vi "Read DMM - Current Mode.vi"(8 "error in (no error)":errorcluster, 11 "Async Data in":T1={"Hardware"={"Switch Device"="", "DMM Device"="", "DMM -> Switch Trigger"=0, "Switch -> DMM Trigger"=0, "Sample Interval (sec)"=0.0, "Current Samples"=0, "Current Limit"=1.2, "Current Resolution"=5.5, "Auto-Read"=FALSE, "Keep Values"=FALSE}, "Communication"={"Status Q"=refnum, "Command Q"=refnum, "Voltage FIFO"=refnum, "Voltage Buffer"=[], "Current FIFO"=refnum, "Current Buffer"=[], "Async Events"=refnum}} {"Hardware"."Current Resolution" items=["3 1/2"=3.5, "4 1/2"=4.5, "5 1/2"=5.5, "6 1/2"=6.5, "7 1/2"=7.5]; "Hardware"."Sample Interval (sec)" format="%.2f"}) -> (0 "error out":errorcluster, 3 "Acquiring":bool)   [LabVIEW 2011, in "Switch-DMM Custom Device.lvlib"]
uses:
  Switch-DMM Custom Device.lvlib
  Controls/Async Data.ctl
  Controls/Hardware.ctl
  <instrlib>/niDMM/nidmm.llb/niDMM Resolution in Digits.ctl
  Controls/Communication.ctl
  Controls/Async Status.ctl
  Controls/Async State.ctl
  Controls/Async Command.ctl
  Controls/Async Events.ctl
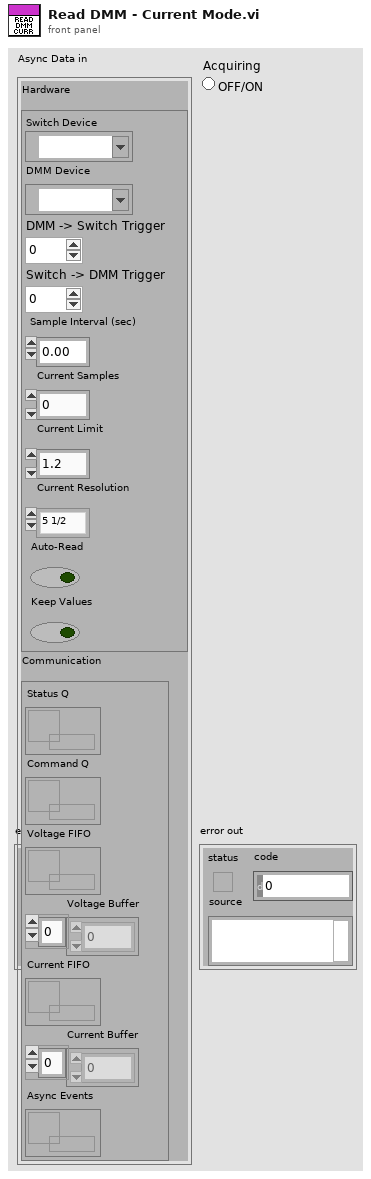
[diagram p1: front panel]
types:
  T1 = typedef "Switch-DMM Custom Device.lvlib/Async Data.ctl" = cluster{"Hardware":T2, "Communication":T4}
  T2 = typedef "Switch-DMM Custom Device.lvlib/Hardware.ctl" = cluster{"Switch Device":refnum<k15>, "DMM Device":refnum<k15>, "DMM -> Switch Trigger":u16, "Switch -> DMM Trigger":u16, "Sample Interval (sec)":dbl, "Current Samples":i32, "Current Limit":dbl, "Current Resolution":T3, "Auto-Read":bool, "Keep Values":bool}
  T3 = typedef "niDMM Resolution in Digits.ctl" = dbl
  T4 = typedef "Switch-DMM Custom Device.lvlib/Communication.ctl" = cluster{"Status Q":refnum<queue>, "Command Q":refnum<queue>, "Voltage FIFO":refnum<k33>, "Voltage Buffer":dbl[], "Current FIFO":refnum<k33>, "Current Buffer":dbl[], "Async Events":refnum<queue>}
  T5 = typedef "Switch-DMM Custom Device.lvlib/Async Events.ctl" = enum16{"None", "Over Current", "Volt Read Done"}
  T6 = typedef "Switch-DMM Custom Device.lvlib/Async Command.ctl" = enum16{"None", "Start", "Set Cur Mode", "Req Volt Mode", "Set Volt Mode", "Read Volt", "Exit"}
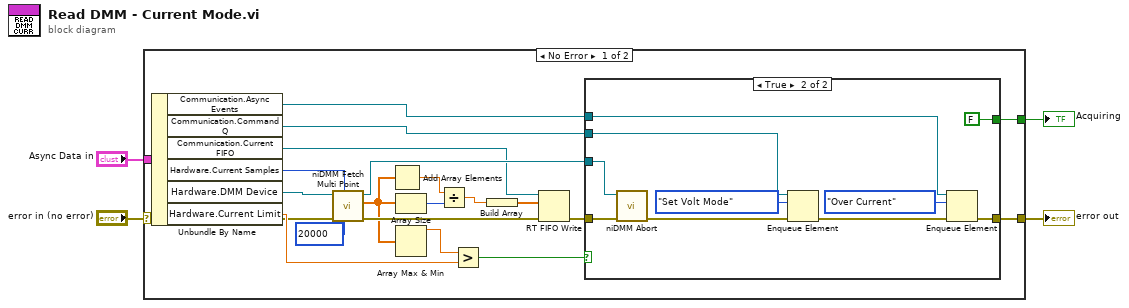
[diagram p0: block diagram]
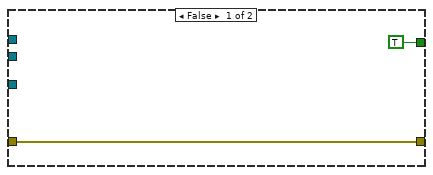
[diagram p2: hidden frame]
diagram:
  n1 = case shown="No Error" "error in (no error)" {
    selector: "error in (no error)" -> [w15 w38]
    tunnel: [w21 w38] -> w4
    tunnel: [w20 _] -> w3
    tunnel: "Async Data in" -> [w16 _]
    frame No Error {
      n2 = Unbundle By Name(w16) -> ("Communication.Async Events"=w13:refnum<queue>, "Communication.Command Q"=w14:refnum<queue>, "Communication.Current FIFO"=w12:refnum<k33>, "Hardware.Current Samples"=w11:i32, "Hardware.DMM Device"=w19:refnum<k15>, "Hardware.Current Limit"=w22:dbl)
      n3 = call <instrlib>:"niDMM Fetch Multi Point.vi"("Maximum Time (msec)"=20000, "Number to Fetch"=w11, "error in (no error)"=w15, "instrument handle"=w19) -> ("error out"=w24:errorcluster, "Measurements"=w8:dbl[], "instrument handle out"=w23:refnum<k15>)  [unwired: 4 in, 1 out]
      n4 = Add Array Elements(numeric array=w8) -> (sum=w9:dbl)
      n5 = Array Size(array=w8) -> (size(s)=w7:i32)
      n6 = Array Max & Min(array=w8) -> (max value=w10:dbl)  [unwired: 3 out]
      n7 = Divide(x=w9, y=w7) -> (x/y=w6:dbl)
      n8 = Greater?(x=w10, y=w22) -> (0:w17:bool)
      n9 = Build Array(w6) -> (w5:dbl[])
      n10 = RT FIFO Write(0:w12, 1:w5, 3:w24) -> (11:w25:errorcluster)  [unwired: 2 in, 3 out]
      n11 = case shown="True" w17 {
        tunnel: w14 -> [_ w37]
        tunnel: [TRUE FALSE] -> w20
        tunnel: w25 -> [w27 w33]
        tunnel: [w27 w29] -> w21
        tunnel: w23 -> [_ w34]
        tunnel: w13 -> [_ w31]
        frame False {
        }
        frame True {
          n12 = call <instrlib>:"niDMM Abort.vi"("error in (no error)"=w33, "instrument handle"=w34) -> ("error out"=w28:errorcluster)  [unwired: 8 in, 1 out]
          n13 = Enqueue Element(queue=w37, element=Async_Command."Set Volt Mode", error in (no error)=w28) -> (error out=w32:errorcluster)  [unwired: 1 in, 2 out]
          n14 = Enqueue Element(queue=w31, element=Async_Events."Over Current", error in (no error)=w32) -> (error out=w29:errorcluster)  [unwired: 1 in, 2 out]
        }
      }
    }
    frame Error {
    }
  }
  "error out" <- w4
  "Acquiring" <- w3
